vi "To Serial Form.vi"(6 "Serial Version":T1, 10 "Serializer in":refnum<class "Serializer.lvclass">, 11 "M data in":refnum<class "M data.lvclass">) -> (0 "error out":errorcluster, 2 "Serializer out":refnum<class "Serializer.lvclass">, 3 "M data out":refnum<class "M data.lvclass">)   [LabVIEW 2014, in "M data.lvclass"]
uses:
  M data.lvclass
  <vilib>/NI/AQ Character Lineator/Serializer/Serializer.lvclass
  <vilib>/NI/AQ Character Lineator/Serialization Common/Serial Version.ctl
  M data.lvclass/M data.ctl
  <vilib>/NI/AQ Character Lineator/Serializable/Insert Single.vi
  <vilib>/NI/AQ Character Lineator/Serializer/Insert Single.vi
  <vilib>/NI/AQ Character Lineator/Serializer/Read Include Default Values.vi
  Alicat Data.lvclass
  <vilib>/NI/AQ Character Lineator/Serializable/Serializable.lvclass
  <vilib>/NI/AQ Character Lineator/Serialization Common/Serialization Common.lvlib
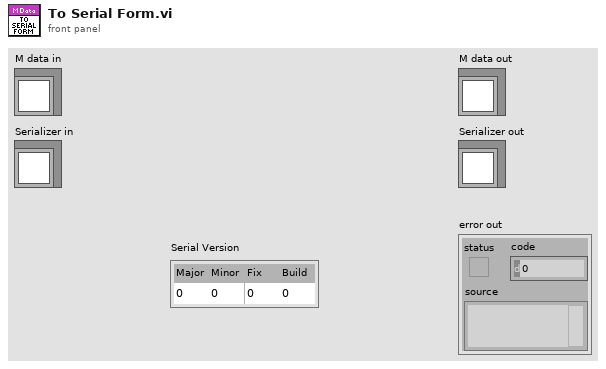
[diagram p1: front panel]
types:
  T1 = typedef "Serialization Common.lvlib/Serial Version.ctl" = cluster{"Major":u16, "Minor":u16, "Fix":u16, "Build":u16}
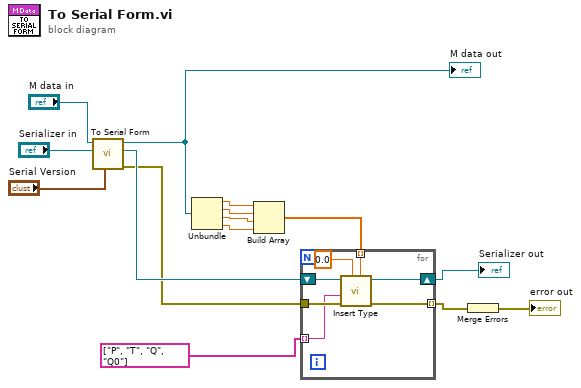
[diagram p0: block diagram]
diagram:
  n1 = call-parent "To Serial Form.vi"("Serial Version"="Serial Version", "Serializer in"="Serializer in", "Data in"="M data in") -> ("error out"=w11:errorcluster, "Serializer out"=w12:refnum<class "Serializer.lvclass">, "Data out"=w10:refnum<class "M data.lvclass">)  [unwired: 6 in]
  "M data out" <- w10
  n2 = Unbundle(w10) -> (w9:sgl, w8:sgl, w7:sgl, w6:sgl)
  n3 = Build Array(w9, w8, w7, w6) -> (w5:sgl[])
  n4 = for {
    tunnel: w11 -> [w21]
    tunnel: w5 -> [w20] mode=indexing
    tunnel: string[] ["P", "T", "Q", "Q0"] -> [w18] mode=indexing
    shift-right: [w17] -> w3
    shift-left: w12 -> [w22]
    tunnel: [w16] -> w2 mode=indexing
    n5 = call-poly <vilib>:"Insert Type.vi"("Double"=w20, "Default Value"=sgl 0.0, "error in (no error)"=w21, "Name"=w18, "Serializer in"=w22) -> ("error out"=w16:errorcluster, "Serializer out"=w17:refnum<class "Serializer.lvclass">)  [unwired: 5 in]
  }
  "Serializer out" <- w3
  n6 = Merge Errors(w2) -> (→"error out":errorcluster)
